vi "NTCP Connected DAO.vi"(8 "error in (no error)":errorcluster, 9 "NTCP Connected In":bool, 11 "DAO Actions":T1=enum."Get") -> (0 "error out":errorcluster, 1 "NTCP Connected Out":bool)   [LabVIEW 2009]
uses:
  Data Access Objects/Metadata/DAO Actions.ctl
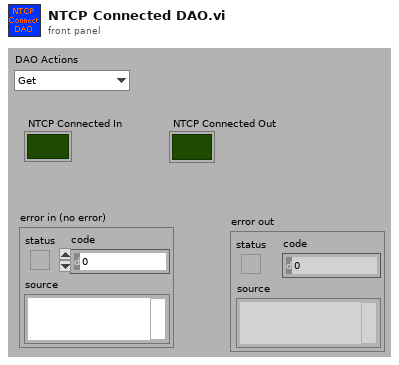
[diagram p1: front panel]
types:
  T1 = typedef "DAO Actions.ctl" = enum16{"Init", "Get", "Set"}
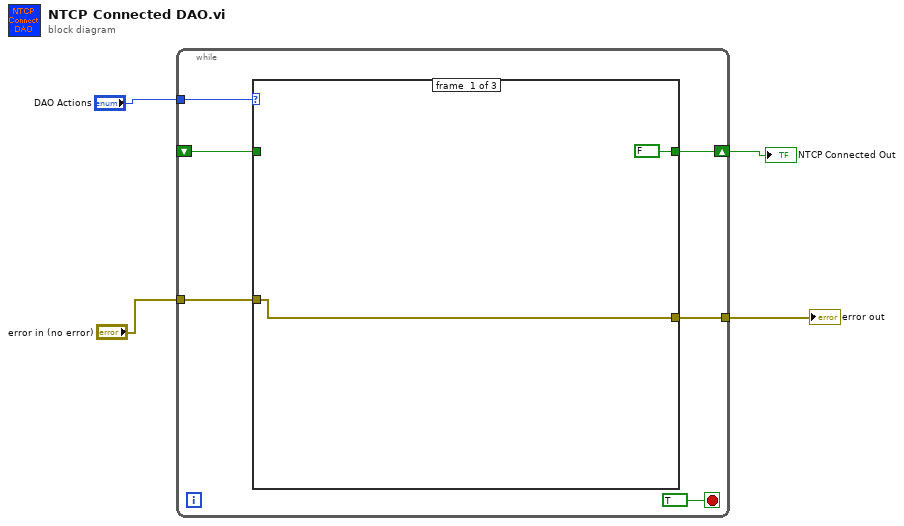
[diagram p0: block diagram]
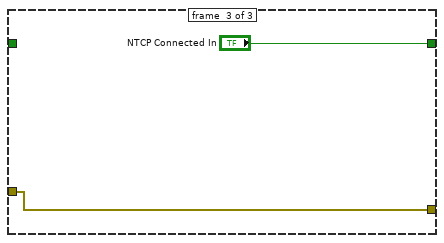
[diagram p3: hidden frame]
diagram:
  n1 = while {
    tunnel: "DAO Actions" -> [w10]
    tunnel: "error in (no error)" -> [w9]
    shift-right: [w8] -> w2
    shift-left: _ -> [w7]
    tunnel: [w5] -> w1
    stop <- TRUE stop-if-true
    n2 = case shown="\"Set\"" w10 {
      tunnel: w9 -> [w11 w13 w15]
      tunnel: [FALSE w14 "NTCP Connected In"] -> w8
      tunnel: w7 -> [_ w14 _]
      tunnel: [w11 w13 w15] -> w5
      frame #0 {
      }
      frame #1 {
      }
      frame #2 {
      }
    }
  }
  "NTCP Connected Out" <- w2
  "error out" <- w1
